vi "ProfilerTest.vi"() -> ()   [LabVIEW 2014] (continued)
"delVelocity"=0.0}, {"Time"=11.409999999999801, "delVelocity"=0.0}, {"Time"=11.419999999999801, "delVelocity"=0.0}, {"Time"=11.4299999999998, "delVelocity"=0.0}, {"Time"=11.4399999999998, "delVelocity"=0.0}, {"Time"=11.4499999999998, "delVelocity"=0.0}, {"Time"=11.4599999999998, "delVelocity"=0.0}, {"Time"=11.4699999999998, "delVelocity"=0.0}, {"Time"=11.4799999999998, "delVelocity"=0.0}, {"Time"=11.4899999999998, "delVelocity"=0.0}, {"Time"=11.4999999999998, "delVelocity"=0.0}, {"Time"=11.509999999999799, "delVelocity"=0.0}, {"Time"=11.519999999999799, "delVelocity"=0.0}, {"Time"=11.529999999999799, "delVelocity"=0.0}, {"Time"=11.539999999999798, "delVelocity"=0.0}, {"Time"=11.549999999999798, "delVelocity"=0.0}, {"Time"=11.559999999999798, "delVelocity"=0.0}, {"Time"=11.569999999999798, "delVelocity"=0.0}, {"Time"=11.579999999999798, "delVelocity"=0.0}, {"Time"=11.589999999999797, "delVelocity"=0.0}, {"Time"=11.599999999999797, "delVelocity"=0.0}, {"Time"=11.609999999999797, "delVelocity"=0.0}, {"Time"=11.619999999999797, "delVelocity"=0.0}, {"Time"=11.629999999999797, "delVelocity"=0.0}, {"Time"=11.639999999999796, "delVelocity"=0.0}, {"Time"=11.649999999999796, "delVelocity"=0.0}, {"Time"=11.659999999999796, "delVelocity"=0.0}, {"Time"=11.669999999999796, "delVelocity"=0.0}, {"Time"=11.679999999999795, "delVelocity"=0.0}, {"Time"=11.689999999999795, "delVelocity"=0.0}, {"Time"=11.699999999999795, "delVelocity"=0.0}, {"Time"=11.709999999999795, "delVelocity"=0.0}, {"Time"=11.719999999999795, "delVelocity"=0.0}, {"Time"=11.729999999999794, "delVelocity"=0.0}, {"Time"=11.739999999999794, "delVelocity"=0.0}, {"Time"=11.749999999999794, "delVelocity"=0.0}, {"Time"=11.759999999999794, "delVelocity"=0.0}, {"Time"=11.769999999999794, "delVelocity"=0.0}, {"Time"=11.779999999999793, "delVelocity"=0.0}, {"Time"=11.789999999999793, "delVelocity"=0.0}, {"Time"=11.799999999999793, "delVelocity"=0.0}, {"Time"=11.809999999999793, "delVelocity"=0.0}, {"Time"=11.819999999999792, "delVelocity"=0.0}, {"Time"=11.829999999999792, "delVelocity"=0.0}, {"Time"=11.839999999999792, "delVelocity"=0.0}, {"Time"=11.849999999999792, "delVelocity"=0.0}, {"Time"=11.859999999999792, "delVelocity"=0.0}, {"Time"=11.869999999999791, "delVelocity"=0.0}, {"Time"=11.879999999999791, "delVelocity"=0.0}, {"Time"=11.889999999999791, "delVelocity"=0.0}, {"Time"=11.89999999999979, "delVelocity"=0.0}, {"Time"=11.90999999999979, "delVelocity"=0.0}, {"Time"=11.91999999999979, "delVelocity"=0.0}, {"Time"=11.92999999999979, "delVelocity"=0.0}, {"Time"=11.93999999999979, "delVelocity"=0.0}, {"Time"=11.94999999999979, "delVelocity"=0.0}, {"Time"=11.95999999999979, "delVelocity"=0.0}, {"Time"=11.96999999999979, "delVelocity"=0.0}, {"Time"=11.979999999999789, "delVelocity"=0.0}, {"Time"=11.989999999999789, "delVelocity"=0.0}, {"Time"=11.999999999999789, "delVelocity"=0.0}, {"Time"=12.009999999999788, "delVelocity"=0.0}, {"Time"=12.019999999999788, "delVelocity"=0.0}, {"Time"=12.029999999999788, "delVelocity"=0.0}, {"Time"=12.039999999999788, "delVelocity"=0.0}, {"Time"=12.049999999999788, "delVelocity"=0.0}, {"Time"=12.059999999999787, "delVelocity"=0.0}, {"Time"=12.069999999999787, "delVelocity"=0.0}, {"Time"=12.079999999999787, "delVelocity"=0.0}, {"Time"=12.089999999999787, "delVelocity"=0.0}, {"Time"=12.099999999999786, "delVelocity"=0.0}, {"Time"=12.109999999999786, "delVelocity"=0.0}, {"Time"=12.119999999999786, "delVelocity"=0.0}, {"Time"=12.129999999999786, "delVelocity"=0.0}, {"Time"=12.139999999999786, "delVelocity"=0.0}, {"Time"=12.149999999999785, "delVelocity"=0.0}, {"Time"=12.159999999999785, "delVelocity"=0.0}, {"Time"=12.169999999999785, "delVelocity"=0.0}, {"Time"=12.179999999999785, "delVelocity"=0.0}, {"Time"=12.189999999999785, "delVelocity"=0.0}, {"Time"=12.199999999999784, "delVelocity"=0.0}, {"Time"=12.209999999999784, "delVelocity"=0.0}, {"Time"=12.219999999999784, "delVelocity"=0.0}, {"Time"=12.229999999999784, "delVelocity"=0.0}, {"Time"=12.239999999999783, "delVelocity"=0.0}, {"Time"=12.249999999999783, "delVelocity"=0.0}, {"Time"=12.259999999999783, "delVelocity"=0.0}, {"Time"=12.269999999999783, "delVelocity"=0.0}, {"Time"=12.279999999999783, "delVelocity"=0.0}, {"Time"=12.289999999999782, "delVelocity"=0.0}, {"Time"=12.299999999999782, "delVelocity"=0.0}, {"Time"=12.309999999999782, "delVelocity"=0.0}, {"Time"=12.319999999999782, "delVelocity"=0.0}, {"Time"=12.329999999999782, "delVelocity"=0.0}, {"Time"=12.339999999999781, "delVelocity"=0.0}, {"Time"=12.349999999999781, "delVelocity"=0.0}, {"Time"=12.359999999999781, "delVelocity"=0.0}, {"Time"=12.36999999999978, "delVelocity"=0.0}, {"Time"=12.37999999999978, "delVelocity"=0.0}, {"Time"=12.38999999999978, "delVelocity"=0.0}, {"Time"=12.39999999999978, "delVelocity"=0.0}, {"Time"=12.40999999999978, "delVelocity"=0.0}, {"Time"=12.41999999999978, "delVelocity"=0.0}, {"Time"=12.42999999999978, "delVelocity"=0.0}, {"Time"=12.43999999999978, "delVelocity"=0.0}, {"Time"=12.449999999999779, "delVelocity"=0.0}, {"Time"=12.459999999999779, "delVelocity"=0.0}, {"Time"=12.469999999999779, "delVelocity"=0.0}, {"Time"=12.479999999999778, "delVelocity"=0.0}, {"Time"=12.489999999999778, "delVelocity"=0.0}, {"Time"=12.499999999999778, "delVelocity"=0.0}, {"Time"=12.509999999999778, "delVelocity"=0.0}, {"Time"=12.519999999999778, "delVelocity"=0.0}, {"Time"=12.529999999999777, "delVelocity"=0.0}, {"Time"=12.539999999999777, "delVelocity"=0.0}, {"Time"=12.549999999999777, "delVelocity"=0.0}, {"Time"=12.559999999999777, "delVelocity"=0.0}, {"Time"=12.569999999999776, "delVelocity"=0.0}, {"Time"=12.579999999999776, "delVelocity"=0.0}, {"Time"=12.589999999999776, "delVelocity"=0.0}, {"Time"=12.599999999999776, "delVelocity"=0.0}, {"Time"=12.609999999999776, "delVelocity"=0.0}, {"Time"=12.619999999999775, "delVelocity"=0.0}, {"Time"=12.629999999999775, "delVelocity"=0.0}, {"Time"=12.639999999999775, "delVelocity"=0.0}, {"Time"=12.649999999999775, "delVelocity"=0.0}, {"Time"=12.659999999999775, "delVelocity"=0.0}, {"Time"=12.669999999999774, "delVelocity"=0.0}, {"Time"=12.679999999999774, "delVelocity"=0.0}, {"Time"=12.689999999999774, "delVelocity"=0.0}, {"Time"=12.699999999999774, "delVelocity"=0.0}, {"Time"=12.709999999999773, "delVelocity"=0.0}, {"Time"=12.719999999999773, "delVelocity"=0.0}, {"Time"=12.729999999999773, "delVelocity"=0.0}, {"Time"=12.739999999999773, "delVelocity"=0.0}, {"Time"=12.749999999999773, "delVelocity"=0.0}, {"Time"=12.759999999999772, "delVelocity"=0.0}, {"Time"=12.769999999999772, "delVelocity"=0.0}, {"Time"=12.779999999999772, "delVelocity"=0.0}, {"Time"=12.789999999999772, "delVelocity"=0.0}, {"Time"=12.799999999999772, "delVelocity"=0.0}, {"Time"=12.809999999999771, "delVelocity"=0.0}, {"Time"=12.819999999999771, "delVelocity"=0.0}, {"Time"=12.829999999999771, "delVelocity"=0.0}, {"Time"=12.83999999999977, "delVelocity"=0.0}, {"Time"=12.84999999999977, "delVelocity"=0.0}, {"Time"=12.85999999999977, "delVelocity"=0.0}, {"Time"=12.86999999999977, "delVelocity"=0.0}, {"Time"=12.87999999999977, "delVelocity"=0.0}, {"Time"=12.88999999999977, "delVelocity"=0.0}, {"Time"=12.89999999999977, "delVelocity"=0.0}, {"Time"=12.90999999999977, "delVelocity"=0.0}, {"Time"=12.919999999999769, "delVelocity"=0.0}, {"Time"=12.929999999999769, "delVelocity"=0.0}, {"Time"=12.939999999999769, "delVelocity"=0.0}, {"Time"=12.949999999999768, "delVelocity"=0.0}, {"Time"=12.959999999999768, "delVelocity"=0.0}, {"Time"=12.969999999999768, "delVelocity"=0.0}, {"Time"=12.979999999999768, "delVelocity"=0.0}, {"Time"=12.989999999999768, "delVelocity"=0.0}, {"Time"=12.999999999999767, "delVelocity"=0.0}, {"Time"=13.009999999999767, "delVelocity"=0.0}, {"Time"=13.019999999999767, "delVelocity"=0.0}, {"Time"=13.029999999999767, "delVelocity"=0.0}, {"Time"=13.039999999999766, "delVelocity"=0.0}, {"Time"=13.049999999999766, "delVelocity"=0.0}, {"Time"=13.059999999999766, "delVelocity"=0.0}, {"Time"=13.069999999999766, "delVelocity"=0.0}, {"Time"=13.079999999999766, "delVelocity"=0.0}, {"Time"=13.089999999999765, "delVelocity"=0.0}, {"Time"=13.099999999999765, "delVelocity"=0.0}, {"Time"=13.109999999999765, "delVelocity"=0.0}, {"Time"=13.119999999999765, "delVelocity"=0.0}, {"Time"=13.129999999999765, "delVelocity"=0.0}, {"Time"=13.139999999999764, "delVelocity"=0.0}, {"Time"=13.149999999999764, "delVelocity"=0.0}, {"Time"=13.159999999999764, "delVelocity"=0.0}, {"Time"=13.169999999999764, "delVelocity"=0.0}, {"Time"=13.179999999999763, "delVelocity"=0.0}, {"Time"=13.189999999999763, "delVelocity"=0.0}, {"Time"=13.199999999999763, "delVelocity"=0.0}, {"Time"=13.209999999999763, "delVelocity"=0.0}, {"Time"=13.219999999999763, "delVelocity"=0.0}, {"Time"=13.229999999999762, "delVelocity"=0.0}, {"Time"=13.239999999999762, "delVelocity"=0.0}, {"Time"=13.249999999999762, "delVelocity"=0.0}, {"Time"=13.259999999999762, "delVelocity"=0.0}, {"Time"=13.269999999999762, "delVelocity"=0.0}, {"Time"=13.279999999999761, "delVelocity"=0.0}, {"Time"=13.289999999999761, "delVelocity"=0.0}, {"Time"=13.299999999999761, "delVelocity"=0.0}, {"Time"=13.30999999999976, "delVelocity"=0.0}, {"Time"=13.31999999999976, "delVelocity"=0.0}, {"Time"=13.32999999999976, "delVelocity"=0.0}, {"Time"=13.33999999999976, "delVelocity"=0.0}, {"Time"=13.34999999999976, "delVelocity"=0.0}, {"Time"=13.35999999999976, "delVelocity"=0.0}, {"Time"=13.36999999999976, "delVelocity"=0.0}, {"Time"=13.37999999999976, "delVelocity"=0.0}, {"Time"=13.389999999999759, "delVelocity"=0.0}, {"Time"=13.399999999999759, "delVelocity"=0.0}, {"Time"=13.409999999999759, "delVelocity"=0.0}, {"Time"=13.419999999999758, "delVelocity"=0.0}, {"Time"=13.429999999999758, "delVelocity"=0.0}, {"Time"=13.439999999999758, "delVelocity"=0.0}, {"Time"=13.449999999999758, "delVelocity"=0.0}, {"Time"=13.459999999999757, "delVelocity"=0.0}, {"Time"=13.469999999999757, "delVelocity"=0.0}, {"Time"=13.479999999999757, "delVelocity"=0.0}, {"Time"=13.489999999999757, "delVelocity"=0.0}, {"Time"=13.499999999999757, "delVelocity"=0.0}, {"Time"=13.509999999999756, "delVelocity"=0.0}, {"Time"=13.519999999999756, "delVelocity"=0.0}, {"Time"=13.529999999999756, "delVelocity"=0.0}, {"Time"=13.539999999999756, "delVelocity"=0.0}, {"Time"=13.549999999999756, "delVelocity"=0.0}, {"Time"=13.559999999999755, "delVelocity"=0.0}, {"Time"=13.569999999999755, "delVelocity"=0.0}, {"Time"=13.579999999999755, "delVelocity"=0.0}, {"Time"=13.589999999999755, "delVelocity"=0.0}, {"Time"=13.599999999999755, "delVelocity"=0.0}, {"Time"=13.609999999999754, "delVelocity"=0.0}, {"Time"=13.619999999999754, "delVelocity"=0.0}, {"Time"=13.629999999999754, "delVelocity"=0.0}, {"Time"=13.639999999999754, "delVelocity"=0.0}, {"Time"=13.649999999999753, "delVelocity"=0.0}, {"Time"=13.659999999999753, "delVelocity"=0.0}, {"Time"=13.669999999999753, "delVelocity"=0.0}, {"Time"=13.679999999999753, "delVelocity"=0.0}, {"Time"=13.689999999999753, "delVelocity"=0.0}, {"Time"=13.699999999999752, "delVelocity"=0.0}, {"Time"=13.709999999999752, "delVelocity"=0.0}, {"Time"=13.719999999999752, "delVelocity"=0.0}, {"Time"=13.729999999999752, "delVelocity"=0.0}, {"Time"=13.739999999999752, "delVelocity"=0.0}, {"Time"=13.749999999999751, "delVelocity"=0.0}, {"Time"=13.759999999999751, "delVelocity"=0.0}, {"Time"=13.76999999999975, "delVelocity"=0.0}, {"Time"=13.77999999999975, "delVelocity"=0.0}, {"Time"=13.78999999999975, "delVelocity"=0.0}, {"Time"=13.79999999999975, "delVelocity"=0.0}, {"Time"=13.80999999999975, "delVelocity"=0.0}, {"Time"=13.81999999999975, "delVelocity"=0.0}, {"Time"=13.82999999999975, "delVelocity"=0.0}, {"Time"=13.83999999999975, "delVelocity"=0.0}, {"Time"=13.84999999999975, "delVelocity"=0.0}, {"Time"=13.859999999999749, "delVelocity"=0.0}, {"Time"=13.869999999999749, "delVelocity"=0.0}, {"Time"=13.879999999999749, "delVelocity"=0.0}, {"Time"=13.889999999999748, "delVelocity"=0.0}, {"Time"=13.899999999999748, "delVelocity"=0.0}, {"Time"=13.909999999999748, "delVelocity"=0.0}, {"Time"=13.919999999999748, "delVelocity"=0.0}, {"Time"=13.929999999999747, "delVelocity"=0.0}, {"Time"=13.939999999999747, "delVelocity"=0.0}, {"Time"=13.949999999999747, "delVelocity"=0.0}, {"Time"=13.959999999999747, "delVelocity"=0.0}, {"Time"=13.969999999999747, "delVelocity"=0.0}, {"Time"=13.979999999999746, "delVelocity"=0.0}, {"Time"=13.989999999999746, "delVelocity"=0.0}, {"Time"=13.999999999999746, "delVelocity"=0.0}, {"Time"=14.009999999999746, "delVelocity"=0.0}, {"Time"=14.019999999999746, "delVelocity"=0.0}, {"Time"=14.029999999999745, "delVelocity"=0.0}, {"Time"=14.039999999999745, "delVelocity"=0.0}, {"Time"=14.049999999999745, "delVelocity"=0.0}, {"Time"=14.059999999999745, "delVelocity"=0.0}, {"Time"=14.069999999999744, "delVelocity"=0.0}, {"Time"=14.079999999999744, "delVelocity"=0.0}, {"Time"=14.089999999999744, "delVelocity"=0.0}, {"Time"=14.099999999999744, "delVelocity"=0.0}, {"Time"=14.109999999999744, "delVelocity"=0.0}, {"Time"=14.119999999999743, "delVelocity"=0.0}, {"Time"=14.129999999999743, "delVelocity"=0.0}, {"Time"=14.139999999999743, "delVelocity"=0.0}, {"Time"=14.149999999999743, "delVelocity"=0.0}, {"Time"=14.159999999999743, "delVelocity"=0.0}, {"Time"=14.169999999999742, "delVelocity"=0.0}, {"Time"=14.179999999999742, "delVelocity"=0.0}, {"Time"=14.189999999999742, "delVelocity"=0.0}, {"Time"=14.199999999999742, "delVelocity"=0.0}, {"Time"=14.209999999999742, "delVelocity"=0.0}, {"Time"=14.219999999999741, "delVelocity"=0.0}, {"Time"=14.229999999999741, "delVelocity"=0.0}, {"Time"=14.23999999999974, "delVelocity"=0.0}, {"Time"=14.24999999999974, "delVelocity"=0.0}, {"Time"=14.25999999999974, "delVelocity"=0.0}, {"Time"=14.26999999999974, "delVelocity"=0.0}, {"Time"=14.27999999999974, "delVelocity"=0.0}, {"Time"=14.28999999999974, "delVelocity"=0.0}, {"Time"=14.29999999999974, "delVelocity"=0.0}, {"Time"=14.30999999999974, "delVelocity"=0.0}, {"Time"=14.31999999999974, "delVelocity"=0.0}, {"Time"=14.329999999999739, "delVelocity"=0.0}, {"Time"=14.339999999999739, "delVelocity"=0.0}, {"Time"=14.349999999999739, "delVelocity"=0.0}, {"Time"=14.359999999999738, "delVelocity"=0.0}, {"Time"=14.369999999999738, "delVelocity"=0.0}, {"Time"=14.379999999999738, "delVelocity"=0.0}, {"Time"=14.389999999999738, "delVelocity"=0.0}, {"Time"=14.399999999999737, "delVelocity"=0.0}, {"Time"=14.409999999999737, "delVelocity"=0.0}, {"Time"=14.419999999999737, "delVelocity"=0.0}, {"Time"=14.429999999999737, "delVelocity"=0.0}, {"Time"=14.439999999999737, "delVelocity"=0.0}, {"Time"=14.449999999999736, "delVelocity"=0.0}, {"Time"=14.459999999999736, "delVelocity"=0.0}, {"Time"=14.469999999999736, "delVelocity"=0.0}, {"Time"=14.479999999999736, "delVelocity"=0.0}, {"Time"=14.489999999999736, "delVelocity"=0.0}, {"Time"=14.499999999999735, "delVelocity"=0.0}, {"Time"=14.509999999999735, "delVelocity"=0.0}, {"Time"=14.519999999999735, "delVelocity"=0.0}, {"Time"=14.529999999999735, "delVelocity"=0.0}, {"Time"=14.539999999999734, "delVelocity"=0.0}, {"Time"=14.549999999999734, "delVelocity"=0.0}, {"Time"=14.559999999999734, "delVelocity"=0.0}, {"Time"=14.569999999999734, "delVelocity"=0.0}, {"Time"=14.579999999999734, "delVelocity"=0.0}, {"Time"=14.589999999999733, "delVelocity"=0.0}, {"Time"=14.599999999999733, "delVelocity"=0.0}, {"Time"=14.609999999999733, "delVelocity"=0.0}, {"Time"=14.619999999999733, "delVelocity"=0.0}, {"Time"=14.629999999999733, "delVelocity"=0.0}, {"Time"=14.639999999999732, "delVelocity"=0.0}, {"Time"=14.649999999999732, "delVelocity"=0.0}, {"Time"=14.659999999999732, "delVelocity"=0.0}, {"Time"=14.669999999999732, "delVelocity"=0.0}, {"Time"=14.679999999999731, "delVelocity"=0.0}, {"Time"=14.689999999999731, "delVelocity"=0.0}, {"Time"=14.699999999999731, "delVelocity"=0.0}, {"Time"=14.70999999999973, "delVelocity"=0.0}, {"Time"=14.71999999999973, "delVelocity"=0.0}, {"Time"=14.72999999999973, "delVelocity"=0.0}, {"Time"=14.73999999999973, "delVelocity"=0.0}, {"Time"=14.74999999999973, "delVelocity"=0.0}, {"Time"=14.75999999999973, "delVelocity"=0.0}, {"Time"=14.76999999999973, "delVelocity"=0.0}, {"Time"=14.77999999999973, "delVelocity"=0.0}, {"Time"=14.78999999999973, "delVelocity"=0.0}, {"Time"=14.799999999999729, "delVelocity"=0.0}, {"Time"=14.809999999999729, "delVelocity"=0.0}, {"Time"=14.819999999999729, "delVelocity"=0.0}, {"Time"=14.829999999999728, "delVelocity"=0.0}, {"Time"=14.839999999999728, "delVelocity"=0.0}, {"Time"=14.849999999999728, "delVelocity"=0.0}, {"Time"=14.859999999999728, "delVelocity"=0.0}, {"Time"=14.869999999999727, "delVelocity"=0.0}, {"Time"=14.879999999999727, "delVelocity"=0.0}, {"Time"=14.889999999999727, "delVelocity"=0.0}, {"Time"=14.899999999999727, "delVelocity"=0.0}, {"Time"=14.909999999999727, "delVelocity"=0.0}, {"Time"=14.919999999999726, "delVelocity"=0.0}, {"Time"=14.929999999999726, "delVelocity"=0.0}, {"Time"=14.939999999999726, "delVelocity"=0.0}, {"Time"=14.949999999999726, "delVelocity"=0.0}, {"Time"=14.959999999999726, "delVelocity"=0.0}, {"Time"=14.969999999999725, "delVelocity"=0.0}, {"Time"=14.979999999999725, "delVelocity"=0.0}, {"Time"=14.989999999999725, "delVelocity"=0.0}, {"Time"=14.999999999999725, "delVelocity"=0.0}, {"Time"=15.009999999999724, "delVelocity"=0.0}, {"Time"=15.019999999999724, "delVelocity"=0.0}, {"Time"=15.029999999999724, "delVelocity"=0.0}, {"Time"=15.039999999999724, "delVelocity"=0.0}, {"Time"=15.049999999999724, "delVelocity"=0.0}, {"Time"=15.059999999999723, "delVelocity"=0.0}, {"Time"=15.069999999999723, "delVelocity"=0.0}, {"Time"=15.079999999999723, "delVelocity"=0.0}, {"Time"=15.089999999999723, "delVelocity"=0.0}, {"Time"=15.099999999999723, "delVelocity"=0.0}, {"Time"=15.109999999999722, "delVelocity"=0.0}, {"Time"=15.119999999999722, "delVelocity"=0.0}, {"Time"=15.129999999999722, "delVelocity"=0.0}, {"Time"=15.139999999999722, "delVelocity"=0.0}, {"Time"=15.149999999999721, "delVelocity"=0.0}, {"Time"=15.159999999999721, "delVelocity"=0.0}, {"Time"=15.169999999999721, "delVelocity"=0.0}, {"Time"=15.17999999999972, "delVelocity"=0.0}, {"Time"=15.18999999999972, "delVelocity"=0.0}, {"Time"=15.19999999999972, "delVelocity"=0.0}, {"Time"=15.20999999999972, "delVelocity"=0.0}, {"Time"=15.21999999999972, "delVelocity"=0.0}, {"Time"=15.22999999999972, "delVelocity"=0.0}, {"Time"=15.23999999999972, "delVelocity"=0.0}, {"Time"=15.24999999999972, "delVelocity"=0.0}, {"Time"=15.25999999999972, "delVelocity"=0.0}, {"Time"=15.269999999999719, "delVelocity"=0.0}, {"Time"=15.279999999999719, "delVelocity"=0.0}, {"Time"=15.289999999999718, "delVelocity"=0.0}, {"Time"=15.299999999999718, "delVelocity"=0.0}, {"Time"=15.309999999999718, "delVelocity"=0.0}, {"Time"=15.319999999999718, "delVelocity"=0.0}, {"Time"=15.329999999999718, "delVelocity"=0.0}, {"Time"=15.339999999999717, "delVelocity"=0.0}, {"Time"=15.349999999999717, "delVelocity"=0.0}, {"Time"=15.359999999999717, "delVelocity"=0.0}, {"Time"=15.369999999999717, "delVelocity"=0.0}, {"Time"=15.379999999999717, "delVelocity"=0.0}, {"Time"=15.389999999999716, "delVelocity"=0.0}, {"Time"=15.399999999999716, "delVelocity"=0.0}, {"Time"=15.409999999999716, "delVelocity"=0.0}, {"Time"=15.419999999999716, "delVelocity"=0.0}, {"Time"=15.429999999999715, "delVelocity"=0.0}, {"Time"=15.439999999999715, "delVelocity"=0.0}, {"Time"=15.449999999999715, "delVelocity"=0.0}, {"Time"=15.459999999999715, "delVelocity"=0.0}, {"Time"=15.469999999999715, "delVelocity"=0.0}, {"Time"=15.479999999999714, "delVelocity"=0.0}, {"Time"=15.489999999999714, "delVelocity"=0.0}, {"Time"=15.499999999999714, "delVelocity"=0.0}, {"Time"=15.509999999999714, "delVelocity"=0.0}, {"Time"=15.519999999999714, "delVelocity"=0.0}, {"Time"=15.529999999999713, "delVelocity"=0.0}, {"Time"=15.539999999999713, "delVelocity"=0.0}, {"Time"=15.549999999999713, "delVelocity"=0.0}, {"Time"=15.559999999999713, "delVelocity"=0.0}, {"Time"=15.569999999999713, "delVelocity"=0.0}, {"Time"=15.579999999999712, "delVelocity"=0.0}, {"Time"=15.589999999999712, "delVelocity"=0.0}, {"Time"=15.599999999999712, "delVelocity"=0.0}, {"Time"=15.609999999999712, "delVelocity"=0.0}, {"Time"=15.619999999999711, "delVelocity"=0.0}, {"Time"=15.629999999999711, "delVelocity"=0.0}, {"Time"=15.639999999999711, "delVelocity"=0.0}, {"Time"=15.64999999999971, "delVelocity"=0.0}, {"Time"=15.65999999999971, "delVelocity"=0.0}, {"Time"=15.66999999999971, "delVelocity"=0.0}, {"Time"=15.67999999999971, "delVelocity"=0.0}, {"Time"=15.68999999999971, "delVelocity"=0.0}, {"Time"=15.69999999999971, "delVelocity"=0.0}, {"Time"=15.70999999999971, "delVelocity"=0.0}, {"Time"=15.71999999999971, "delVelocity"=0.0}, {"Time"=15.729999999999709, "delVelocity"=0.0}, {"Time"=15.739999999999709, "delVelocity"=0.0}, {"Time"=15.749999999999709, "delVelocity"=0.0}, {"Time"=15.759999999999708, "delVelocity"=0.0}, {"Time"=15.769999999999708, "delVelocity"=0.0}, {"Time"=15.779999999999708, "delVelocity"=0.0}, {"Time"=15.789999999999708, "delVelocity"=0.0}, {"Time"=15.799999999999708, "delVelocity"=0.0}, {"Time"=15.809999999999707, "delVelocity"=0.0}, {"Time"=15.819999999999707, "delVelocity"=0.0}, {"Time"=15.829999999999707, "delVelocity"=0.0}, {"Time"=15.839999999999707, "delVelocity"=0.0}, {"Time"=15.849999999999707, "delVelocity"=0.0}, {"Time"=15.859999999999706, "delVelocity"=0.0}, {"Time"=15.869999999999706, "delVelocity"=0.0}, {"Time"=15.879999999999706, "delVelocity"=0.0}, {"Time"=15.889999999999706, "delVelocity"=0.0}, {"Time"=15.899999999999705, "delVelocity"=0.0}, {"Time"=15.909999999999705, "delVelocity"=0.0}, {"Time"=15.919999999999705, "delVelocity"=0.0}, {"Time"=15.929999999999705, "delVelocity"=0.0}, {"Time"=15.939999999999705, "delVelocity"=0.0}, {"Time"=15.949999999999704, "delVelocity"=0.0}, {"Time"=15.959999999999704, "delVelocity"=0.0}, {"Time"=15.969999999999704, "delVelocity"=0.0}, {"Time"=15.979999999999704, "delVelocity"=0.0}, {"Time"=15.989999999999704, "delVelocity"=0.0}, {"Time"=15.999999999999703, "delVelocity"=0.0}, {"Time"=16.009999999999703, "delVelocity"=0.0}, {"Time"=16.019999999999705, "delVelocity"=0.0}, {"Time"=16.029999999999706, "delVelocity"=0.0}, {"Time"=16.039999999999708, "delVelocity"=0.0}, {"Time"=16.04999999999971, "delVelocity"=0.0}, {"Time"=16.05999999999971, "delVelocity"=0.0}, {"Time"=16.069999999999713, "delVelocity"=0.0}, {"Time"=16.079999999999714, "delVelocity"=0.0}, {"Time"=16.089999999999716, "delVelocity"=0.0}, {"Time"=16.099999999999717, "delVelocity"=0.0}, {"Time"=16.10999999999972, "delVelocity"=0.0}, {"Time"=16.11999999999972, "delVelocity"=0.0}, {"Time"=16.129999999999722, "delVelocity"=0.0}, {"Time"=16.139999999999723, "delVelocity"=0.0}, {"Time"=16.149999999999725, "delVelocity"=0.0}, {"Time"=16.159999999999727, "delVelocity"=0.0}, {"Time"=16.169999999999728, "delVelocity"=0.0}, {"Time"=16.17999999999973, "delVelocity"=0.0}, {"Time"=16.18999999999973, "delVelocity"=0.0}, {"Time"=16.199999999999733, "delVelocity"=0.0}, {"Time"=16.209999999999734, "delVelocity"=0.0}, {"Time"=16.219999999999736, "delVelocity"=0.0}, {"Time"=16.229999999999738, "delVelocity"=0.0}, {"Time"=16.23999999999974, "delVelocity"=0.0}, {"Time"=16.24999999999974, "delVelocity"=0.0}, {"Time"=16.259999999999742, "delVelocity"=0.0}, {"Time"=16.269999999999744, "delVelocity"=0.0}, {"Time"=16.279999999999745, "delVelocity"=0.0}, {"Time"=16.289999999999747, "delVelocity"=0.0}, {"Time"=16.29999999999975, "delVelocity"=0.0}, {"Time"=16.30999999999975, "delVelocity"=0.0}, {"Time"=16.31999999999975, "delVelocity"=0.0}, {"Time"=16.329999999999753, "delVelocity"=0.0}, {"Time"=16.339999999999755, "delVelocity"=0.0}, {"Time"=16.349999999999756, "delVelocity"=0.0}, {"Time"=16.359999999999758, "delVelocity"=0.0}, {"Time"=16.36999999999976, "delVelocity"=0.0}, {"Time"=16.37999999999976, "delVelocity"=0.0}, {"Time"=16.389999999999763, "delVelocity"=0.0}, {"Time"=16.399999999999764, "delVelocity"=0.0}, {"Time"=16.409999999999766, "delVelocity"=0.0}, {"Time"=16.419999999999767, "delVelocity"=0.0}, {"Time"=16.42999999999977, "delVelocity"=0.0}, {"Time"=16.43999999999977, "delVelocity"=0.0}, {"Time"=16.449999999999772, "delVelocity"=0.0}, {"Time"=16.459999999999773, "delVelocity"=0.0}, {"Time"=16.469999999999775, "delVelocity"=0.0}, {"Time"=16.479999999999777, "delVelocity"=0.0}, {"Time"=16.489999999999778, "delVelocity"=0.0}, {"Time"=16.49999999999978, "delVelocity"=0.0}, {"Time"=16.50999999999978, "delVelocity"=0.0}, {"Time"=16.519999999999783, "delVelocity"=0.0}, {"Time"=16.529999999999784, "delVelocity"=0.0}, {"Time"=16.539999999999786, "delVelocity"=0.0}, {"Time"=16.549999999999788, "delVelocity"=0.0}, {"Time"=16.55999999999979, "delVelocity"=0.0}, {"Time"=16.56999999999979, "delVelocity"=0.0}, {"Time"=16.579999999999792, "delVelocity"=0.0}, {"Time"=16.589999999999794, "delVelocity"=0.0}, {"Time"=16.599999999999795, "delVelocity"=0.0}, {"Time"=16.609999999999797, "delVelocity"=0.0}, {"Time"=16.6199999999998, "delVelocity"=0.0}, {"Time"=16.6299999999998, "delVelocity"=0.0}, {"Time"=16.6399999999998, "delVelocity"=0.0}, {"Time"=16.649999999999803, "delVelocity"=0.0}, {"Time"=16.659999999999805, "delVelocity"=0.0}, {"Time"=16.669999999999806, "delVelocity"=0.0}, {"Time"=16.679999999999808, "delVelocity"=0.0}, {"Time"=16.68999999999981, "delVelocity"=0.0}, {"Time"=16.69999999999981, "delVelocity"=0.0}, {"Time"=16.709999999999813, "delVelocity"=0.0}, {"Time"=16.719999999999814, "delVelocity"=0.0}, {"Time"=16.729999999999816, "delVelocity"=0.0}, {"Time"=16.739999999999817, "delVelocity"=0.0}, {"Time"=16.74999999999982, "delVelocity"=0.0}, {"Time"=16.75999999999982, "delVelocity"=0.0}, {"Time"=16.769999999999822, "delVelocity"=0.0}, {"Time"=16.779999999999824, "delVelocity"=0.0}, {"Time"=16.789999999999825, "delVelocity"=0.0}, {"Time"=16.799999999999827, "delVelocity"=0.0}, {"Time"=16.809999999999828, "delVelocity"=0.0}, {"Time"=16.81999999999983, "delVelocity"=0.0}, {"Time"=16.82999999999983, "delVelocity"=0.0}, {"Time"=16.839999999999833, "delVelocity"=0.0}, {"Time"=16.849999999999834, "delVelocity"=0.0}, {"Time"=16.859999999999836, "delVelocity"=0.0}, {"Time"=16.869999999999838, "delVelocity"=0.0}, {"Time"=16.87999999999984, "delVelocity"=0.0}, {"Time"=16.88999999999984, "delVelocity"=0.0}, {"Time"=16.899999999999842, "delVelocity"=0.0}, {"Time"=16.909999999999844, "delVelocity"=0.0}, {"Time"=16.919999999999845, "delVelocity"=0.0}, {"Time"=16.929999999999847, "delVelocity"=0.0}, {"Time"=16.93999999999985, "delVelocity"=0.0}, {"Time"=16.94999999999985, "delVelocity"=0.0}, {"Time"=16.95999999999985, "delVelocity"=0.0}, {"Time"=16.969999999999853, "delVelocity"=0.0}, {"Time"=16.979999999999855, "delVelocity"=0.0}, {"Time"=16.989999999999856, "delVelocity"=0.0}, {"Time"=16.999999999999858, "delVelocity"=0.0}, {"Time"=17.00999999999986, "delVelocity"=0.0}, {"Time"=17.01999999999986, "delVelocity"=0.0}, {"Time"=17.029999999999863, "delVelocity"=0.0}, {"Time"=17.039999999999864, "delVelocity"=0.0}, {"Time"=17.049999999999866, "delVelocity"=0.0}, {"Time"=17.059999999999867, "delVelocity"=0.0}, {"Time"=17.06999999999987, "delVelocity"=0.0}, {"Time"=17.07999999999987, "delVelocity"=0.0}, {"Time"=17.089999999999872, "delVelocity"=0.0}, {"Time"=17.099999999999874, "delVelocity"=0.0}, {"Time"=17.109999999999875, "delVelocity"=0.0}, {"Time"=17.119999999999877, "delVelocity"=0.0}, {"Time"=17.129999999999878, "delVelocity"=0.0}, {"Time"=17.13999999999988, "delVelocity"=0.0}, {"Time"=17.14999999999988, "delVelocity"=0.0}, {"Time"=17.159999999999883, "delVelocity"=0.0}, {"Time"=17.169999999999884, "delVelocity"=0.0}, {"Time"=17.179999999999886, "delVelocity"=0.0}, {"Time"=17.189999999999888, "delVelocity"=0.0}, {"Time"=17.19999999999989, "delVelocity"=0.0}, {"Time"=17.20999999999989, "delVelocity"=0.0}, {"Time"=17.219999999999892, "delVelocity"=0.0}, {"Time"=17.229999999999894, "delVelocity"=0.0}, {"Time"=17.239999999999895, "delVelocity"=0.0}, {"Time"=17.249999999999897, "delVelocity"=0.0}, {"Time"=17.2599999999999, "delVelocity"=0.0}, {"Time"=17.2699999999999, "delVelocity"=0.0}, {"Time"=17.2799999999999, "delVelocity"=0.0}, {"Time"=17.289999999999903, "delVelocity"=0.0}, {"Time"=17.299999999999905, "delVelocity"=0.0}, {"Time"=17.309999999999906, "delVelocity"=0.0}, {"Time"=17.319999999999908, "delVelocity"=0.0}, {"Time"=17.32999999999991, "delVelocity"=0.0}, {"Time"=17.33999999999991, "delVelocity"=0.0}, {"Time"=17.349999999999913, "delVelocity"=0.0}, {"Time"=17.359999999999914, "delVelocity"=0.0}, {"Time"=17.369999999999916, "delVelocity"=0.0}, {"Time"=17.379999999999917, "delVelocity"=0.0}, {"Time"=17.38999999999992, "delVelocity"=0.0}, {"Time"=17.39999999999992, "delVelocity"=0.0}, {"Time"=17.409999999999922, "delVelocity"=0.0}, {"Time"=17.419999999999924, "delVelocity"=0.0}, {"Time"=17.429999999999925, "delVelocity"=0.0}, {"Time"=17.439999999999927, "delVelocity"=0.0}, {"Time"=17.44999999999993, "delVelocity"=0.0}, {"Time"=17.45999999999993, "delVelocity"=0.0}, {"Time"=17.46999999999993, "delVelocity"=0.0}, {"Time"=17.479999999999933, "delVelocity"=0.0}, {"Time"=17.489999999999934, "delVelocity"=0.0}, {"Time"=17.499999999999936, "delVelocity"=0.0}, {"Time"=17.509999999999938, "delVelocity"=0.0}, {"Time"=17.51999999999994, "delVelocity"=0.0}, {"Time"=17.52999999999994, "delVelocity"=0.0}, {"Time"=17.539999999999942, "delVelocity"=0.0}, {"Time"=17.549999999999944, "delVelocity"=0.0}, {"Time"=17.559999999999945, "delVelocity"=0.0}, {"Time"=17.569999999999947, "delVelocity"=0.0}, {"Time"=17.57999999999995, "delVelocity"=0.0}, {"Time"=17.58999999999995, "delVelocity"=0.0}, {"Time"=17.59999999999995, "delVelocity"=0.0}, {"Time"=17.609999999999953, "delVelocity"=0.0}, {"Time"=17.619999999999955, "delVelocity"=0.0}, {"Time"=17.629999999999956, "delVelocity"=0.0}, {"Time"=17.639999999999958, "delVelocity"=0.0}, {"Time"=17.64999999999996, "delVelocity"=0.0}, {"Time"=17.65999999999996, "delVelocity"=0.0}, {"Time"=17.669999999999963, "delVelocity"=0.0}, {"Time"=17.679999999999964, "delVelocity"=0.0}, {"Time"=17.689999999999966, "delVelocity"=0.0}, {"Time"=17.699999999999967, "delVelocity"=0.0}, {"Time"=17.70999999999997, "delVelocity"=0.0}, {"Time"=17.71999999999997, "delVelocity"=0.0}, {"Time"=17.729999999999972, "delVelocity"=0.0}, {"Time"=17.739999999999974, "delVelocity"=0.0}, {"Time"=17.749999999999975, "delVelocity"=0.0}, {"Time"=17.759999999999977, "delVelocity"=0.0}, {"Time"=17.76999999999998, "delVelocity"=0.0}, {"Time"=17.77999999999998, "delVelocity"=0.0}, {"Time"=17.78999999999998, "delVelocity"=0.0}, {"Time"=17.799999999999983, "delVelocity"=0.0}, {"Time"=17.809999999999985, "delVelocity"=0.0}, {"Time"=17.819999999999986, "delVelocity"=0.0}, {"Time"=17.829999999999988, "delVelocity"=0.0}, {"Time"=17.83999999999999, "delVelocity"=0.0}, {"Time"=17.84999999999999, "delVelocity"=0.0}, {"Time"=17.859999999999992, "delVelocity"=0.0}, {"Time"=17.869999999999994, "delVelocity"=0.0}, {"Time"=17.879999999999995, "delVelocity"=0.0}, {"Time"=17.889999999999997, "delVelocity"=0.0}, {"Time"=17.9, "delVelocity"=0.0}, {"Time"=17.91, "delVelocity"=0.0}, {"Time"=17.92, "delVelocity"=0.0}, {"Time"=17.930000000000003, "delVelocity"=0.0}, {"Time"=17.940000000000005, "delVelocity"=0.0}, {"Time"=17.950000000000006, "delVelocity"=0.0}, {"Time"=17.960000000000008, "delVelocity"=0.0}, {"Time"=17.97000000000001, "delVelocity"=0.0}, {"Time"=17.98000000000001, "delVelocity"=0.0}, {"Time"=17.990000000000013, "delVelocity"=0.0}, {"Time"=18.000000000000014, "delVelocity"=0.0}, {"Time"=18.010000000000016, "delVelocity"=0.0}, {"Time"=18.020000000000017, "delVelocity"=0.0}, {"Time"=18.03000000000002, "delVelocity"=0.0}, {"Time"=18.04000000000002, "delVelocity"=0.0}, {"Time"=18.050000000000022, "delVelocity"=0.0}, {"Time"=18.060000000000024, "delVelocity"=0.0}, {"Time"=18.070000000000025, "delVelocity"=0.0}, {"Time"=18.080000000000027, "delVelocity"=0.0}, {"Time"=18.09000000000003, "delVelocity"=0.0}, {"Time"=18.10000000000003, "delVelocity"=0.0}, {"Time"=18.11000000000003, "delVelocity"=0.0}, {"Time"=18.120000000000033, "delVelocity"=0.0}, {"Time"=18.130000000000035, "delVelocity"=0.0}, {"Time"=18.140000000000036, "delVelocity"=0.0}, {"Time"=18.150000000000038, "delVelocity"=0.0}, {"Time"=18.16000000000004, "delVelocity"=0.0}, {"Time"=18.17000000000004, "delVelocity"=0.0}, {"Time"=18.180000000000042, "delVelocity"=0.0}, {"Time"=18.190000000000044, "delVelocity"=0.0}, {"Time"=18.200000000000045, "delVelocity"=0.0}, {"Time"=18.210000000000047, "delVelocity"=0.0}, {"Time"=18.22000000000005, "delVelocity"=0.0}, {"Time"=18.23000000000005, "delVelocity"=0.0}, {"Time"=18.24000000000005, "delVelocity"=0.0}, {"Time"=18.250000000000053, "delVelocity"=0.0}, {"Time"=18.260000000000055, "delVelocity"=0.0}, {"Time"=18.270000000000056, "delVelocity"=0.0}, {"Time"=18.280000000000058, "delVelocity"=0.0}, {"Time"=18.29000000000006, "delVelocity"=0.0}, {"Time"=18.30000000000006, "delVelocity"=0.0}, {"Time"=18.310000000000063, "delVelocity"=0.0}, {"Time"=18.320000000000064, "delVelocity"=0.0}, {"Time"=18.330000000000066, "delVelocity"=0.0}, {"Time"=18.340000000000067, "delVelocity"=0.0}, {"Time"=18.35000000000007, "delVelocity"=0.0}, {"Time"=18.36000000000007, "delVelocity"=0.0}, {"Time"=18.370000000000072, "delVelocity"=0.0}, {"Time"=18.380000000000074, "delVelocity"=0.0}, {"Time"=18.390000000000075, "delVelocity"=0.0}, {"Time"=18.400000000000077, "delVelocity"=0.0}, {"Time"=18.41000000000008, "delVelocity"=0.0}, {"Time"=18.42000000000008, "delVelocity"=0.0}, {"Time"=18.43000000000008, "delVelocity"=0.0}, {"Time"=18.440000000000083, "delVelocity"=0.0}, {"Time"=18.450000000000085, "delVelocity"=0.0}, {"Time"=18.460000000000086, "delVelocity"=0.0}, {"Time"=18.470000000000088, "delVelocity"=0.0}, {"Time"=18.48000000000009, "delVelocity"=0.0}, {"Time"=18.49000000000009, "delVelocity"=0.0}, {"Time"=18.500000000000092, "delVelocity"=0.0}, {"Time"=18.510000000000094, "delVelocity"=0.0}, {"Time"=18.520000000000095, "delVelocity"=0.0}, {"Time"=18.530000000000097, "delVelocity"=0.0}, {"Time"=18.5400000000001, "delVelocity"=0.0}, {"Time"=18.5500000000001, "delVelocity"=0.0}, {"Time"=18.5600000000001, "delVelocity"=0.0}, {"Time"=18.570000000000103, "delVelocity"=0.0}, {"Time"=18.580000000000105, "delVelocity"=0.0}, {"Time"=18.590000000000106, "delVelocity"=0.0}, {"Time"=18.600000000000108, "delVelocity"=0.0}, {"Time"=18.61000000000011, "delVelocity"=0.0}, {"Time"=18.62000000000011, "delVelocity"=0.0}, {"Time"=18.630000000000113, "delVelocity"=0.0}, {"Time"=18.640000000000114, "delVelocity"=0.0}, {"Time"=18.650000000000116, "delVelocity"=0.0}, {"Time"=18.660000000000117, "delVelocity"=0.0}, {"Time"=18.67000000000012, "delVelocity"=0.0}, {"Time"=18.68000000000012, "delVelocity"=0.0}, {"Time"=18.690000000000122, "delVelocity"=0.0}, {"Time"=18.700000000000124, "delVelocity"=0.0}, {"Time"=18.710000000000125, "delVelocity"=0.0}, {"Time"=18.720000000000127, "delVelocity"=0.0}, {"Time"=18.73000000000013, "delVelocity"=0.0}, {"Time"=18.74000000000013, "delVelocity"=0.0}, {"Time"=18.75000000000013, "delVelocity"=0.0}, {"Time"=18.760000000000133, "delVelocity"=0.0}, {"Time"=18.770000000000135, "delVelocity"=0.0}, {"Time"=18.780000000000136, "delVelocity"=0.0}, {"Time"=18.790000000000138, "delVelocity"=0.0}, {"Time"=18.80000000000014, "delVelocity"=0.0}, {"Time"=18.81000000000014, "delVelocity"=0.0}, {"Time"=18.820000000000142, "delVelocity"=0.0}, {"Time"=18.830000000000144, "delVelocity"=0.0}, {"Time"=18.840000000000146, "delVelocity"=0.0}, {"Time"=18.850000000000147, "delVelocity"=0.0}, {"Time"=18.86000000000015, "delVelocity"=0.0}, {"Time"=18.87000000000015, "delVelocity"=0.0}, {"Time"=18.88000000000015, "delVelocity"=0.0}, {"Time"=18.890000000000153, "delVelocity"=0.0}, {"Time"=18.900000000000155, "delVelocity"=0.0}, {"Time"=18.910000000000156, "delVelocity"=0.0}, {"Time"=18.920000000000158, "delVelocity"=0.0}, {"Time"=18.93000000000016, "delVelocity"=0.0}, {"Time"=18.94000000000016, "delVelocity"=0.0}, {"Time"=18.950000000000163, "delVelocity"=0.0}, {"Time"=18.960000000000164, "delVelocity"=0.0}, {"Time"=18.970000000000166, "delVelocity"=0.0}, {"Time"=18.980000000000167, "delVelocity"=0.0}, {"Time"=18.99000000000017, "delVelocity"=0.0}, {"Time"=19.00000000000017, "delVelocity"=0.0}, {"Time"=19.010000000000172, "delVelocity"=0.0}, {"Time"=19.020000000000174, "delVelocity"=0.0}, {"Time"=19.030000000000175, "delVelocity"=0.0}, {"Time"=19.040000000000177, "delVelocity"=0.0}, {"Time"=19.05000000000018, "delVelocity"=0.0}, {"Time"=19.06000000000018, "delVelocity"=0.0}, {"Time"=19.07000000000018, "delVelocity"=0.0}, {"Time"=19.080000000000183, "delVelocity"=0.0}, {"Time"=19.090000000000185, "delVelocity"=0.0}, {"Time"=19.100000000000186, "delVelocity"=0.0}, {"Time"=19.110000000000188, "delVelocity"=0.0}, {"Time"=19.12000000000019, "delVelocity"=0.0}, {"Time"=19.13000000000019, "delVelocity"=0.0}, {"Time"=19.140000000000192, "delVelocity"=0.0}, {"Time"=19.150000000000194, "delVelocity"=0.0}, {"Time"=19.160000000000196, "delVelocity"=0.0}, {"Time"=19.170000000000197, "delVelocity"=0.0}, {"Time"=19.1800000000002, "delVelocity"=0.0}, {"Time"=19.1900000000002, "delVelocity"=0.0}, {"Time"=19.200000000000202, "delVelocity"=0.0}, {"Time"=19.210000000000203, "delVelocity"=0.0}, {"Time"=19.220000000000205, "delVelocity"=0.0}, {"Time"=19.230000000000206, "delVelocity"=0.0}, {"Time"=19.240000000000208, "delVelocity"=0.0}, {"Time"=19.25000000000021, "delVelocity"=0.0}, {"Time"=19.26000000000021, "delVelocity"=0.0}, {"Time"=19.270000000000213, "delVelocity"=0.0}, {"Time"=19.280000000000214, "delVelocity"=0.0}, {"Time"=19.290000000000216, "delVelocity"=0.0}, {"Time"=19.300000000000217, "delVelocity"=0.0}, {"Time"=19.31000000000022, "delVelocity"=0.0}, {"Time"=19.32000000000022, "delVelocity"=0.0}, {"Time"=19.330000000000222, "delVelocity"=0.0}, {"Time"=19.340000000000224, "delVelocity"=0.0}, {"Time"=19.350000000000225, "delVelocity"=0.0}, {"Time"=19.360000000000227, "delVelocity"=0.0}, {"Time"=19.37000000000023, "delVelocity"=0.0}, {"Time"=19.38000000000023, "delVelocity"=0.0}, {"Time"=19.39000000000023, "delVelocity"=0.0}, {"Time"=19.400000000000233, "delVelocity"=0.0}, {"Time"=19.410000000000235, "delVelocity"=0.0}, {"Time"=19.420000000000236, "delVelocity"=0.0}, {"Time"=19.430000000000238, "delVelocity"=0.0}, {"Time"=19.44000000000024, "delVelocity"=0.0}, {"Time"=19.45000000000024, "delVelocity"=0.0}, {"Time"=19.460000000000242, "delVelocity"=0.0}, {"Time"=19.470000000000244, "delVelocity"=0.0}, {"Time"=19.480000000000246, "delVelocity"=0.0}, {"Time"=19.490000000000247, "delVelocity"=0.0}, {"Time"=19.50000000000025, "delVelocity"=0.0}, {"Time"=19.51000000000025, "delVelocity"=0.0}, {"Time"=19.520000000000252, "delVelocity"=0.0}, {"Time"=19.530000000000253, "delVelocity"=0.0}, {"Time"=19.540000000000255, "delVelocity"=0.0}, {"Time"=19.550000000000257, "delVelocity"=0.0}, {"Time"=19.560000000000258, "delVelocity"=0.0}, {"Time"=19.57000000000026, "delVelocity"=0.0}, {"Time"=19.58000000000026, "delVelocity"=0.0}, {"Time"=19.590000000000263, "delVelocity"=0.0}, {"Time"=19.600000000000264, "delVelocity"=0.0}, {"Time"=19.610000000000266, "delVelocity"=0.0}, {"Time"=19.620000000000267, "delVelocity"=0.0}, {"Time"=19.63000000000027, "delVelocity"=0.0}, {"Time"=19.64000000000027, "delVelocity"=0.0}, {"Time"=19.650000000000272, "delVelocity"=0.0}, {"Time"=19.660000000000274, "delVelocity"=0.0}, {"Time"=19.670000000000275, "delVelocity"=0.0}, {"Time"=19.680000000000277, "delVelocity"=0.0}, {"Time"=19.69000000000028, "delVelocity"=0.0}, {"Time"=19.70000000000028, "delVelocity"=0.0}, {"Time"=19.71000000000028, "delVelocity"=0.0}, {"Time"=19.720000000000283, "delVelocity"=0.0}, {"Time"=19.730000000000285, "delVelocity"=0.0}, {"Time"=19.740000000000286, "delVelocity"=0.0}, {"Time"=19.750000000000288, "delVelocity"=0.0}, {"Time"=19.76000000000029, "delVelocity"=0.0}, {"Time"=19.77000000000029, "delVelocity"=0.0}, {"Time"=19.780000000000292, "delVelocity"=0.0}, {"Time"=19.790000000000294, 
